vi "Initialize Pressure Transducers.vi"(4 "manifold b":dbl=-51999.8452035158 format="%#_13g", 5 "tube b":dbl=-5165625.86475965 format="%#_13g", 6 "manifold m":dbl=13009471.549307 format="%#_13g", 7 "tube m":dbl=1292765951.79248 format="%#_13g", 8 "error in":errorcluster, 9 "Sensor sample period (ms)":i32=100, 11 "file path":path) -> (0 "Error Out":errorcluster, 3 "task out":refnum<k21>)   [LabVIEW 2018]
uses:
  <vilib>/DAQmx/create/scale.llb/DAQmx Create Scale (Linear).vi
  <vilib>/DAQmx/create/channels.llb/DAQmx Create Channel (AI-Current-Basic).vi
  <vilib>/DAQmx/configure/timing.llb/DAQmx Timing (Sample Clock).vi
  <vilib>/DAQmx/configure/task.llb/DAQmx Configure Logging (TDMS).vi
  <resource>/objmgr/daqmx.rc
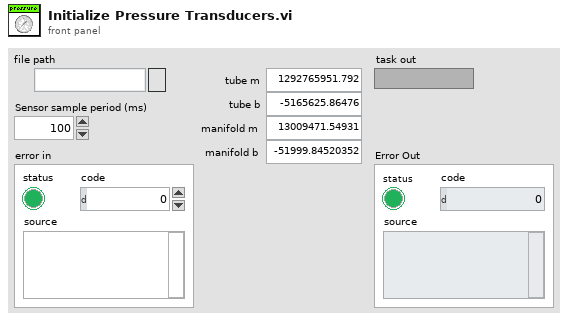
[diagram p1: front panel]
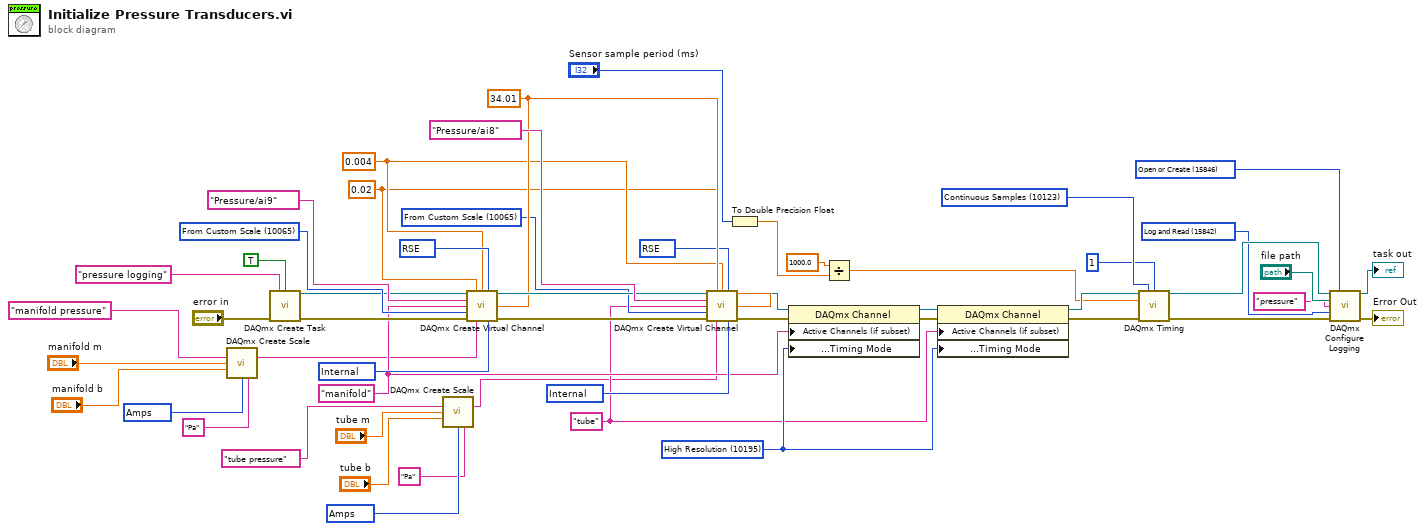
[diagram p0: block diagram]
diagram:
  w10 = 10342 items=["Volts"=10348, "Amps"=10342, "Deg F"=10144, "Deg C"=10143, "Deg R"=10145, "Kelvins"=10325, "Strain"=10299, "Ohms"=10384, "Hz"=10373, "Seconds"=10364, "Meters"=10219, "Inches"=10379, "Degrees"=10146, "Radians"=10273, "Ticks"=10304, "g"=10186, "m/s^2"=12470, "m/s"=15959, "in/s"=15960, "Pascals"=10081, "Newtons"=15875, "Pounds"=15876, "kgf"=15877, "psi"=15879, "bar"=15880, "Nm"=15881, "oz-in"=15882, "lb-in"=15883, "lb-ft"=15884, "Volts/Volt"=15896, "mVolts/Volt"=15897, "pCoulombs"=16103, "Coulombs"=16102, "From TEDS"=12516] ("pre-scaled units")
  w13 = 10342 items=["Volts"=10348, "Amps"=10342, "Deg F"=10144, "Deg C"=10143, "Deg R"=10145, "Kelvins"=10325, "Strain"=10299, "Ohms"=10384, "Hz"=10373, "Seconds"=10364, "Meters"=10219, "Inches"=10379, "Degrees"=10146, "Radians"=10273, "Ticks"=10304, "g"=10186, "m/s^2"=12470, "m/s"=15959, "in/s"=15960, "Pascals"=10081, "Newtons"=15875, "Pounds"=15876, "kgf"=15877, "psi"=15879, "bar"=15880, "Nm"=15881, "oz-in"=15882, "lb-in"=15883, "lb-ft"=15884, "Volts/Volt"=15896, "mVolts/Volt"=15897, "pCoulombs"=16103, "Coulombs"=16102, "From TEDS"=12516] ("pre-scaled units")
  w23 = 15842 items=["Off"=10231, "Log"=15844, "Log and Read"=15842] ("logging mode")
  w24 = 15846 items=["Open"=10437, "Open or Create"=15846, "Create or Replace"=15847, "Create"=15848] ("operation")
  w35 = 10123 items=["Finite Samples"=10178, "Continuous Samples"=10123, "Hardware Timed Single Point"=12522] ("sample mode")
  w38 = 10200 items=["default"=-1, "Internal"=10200, "External"=10167] ("shunt resistor location")
  w39 = 10065 items=["Amps"=10342, "From Custom Scale"=10065] ("units")
  w40 = 10083 items=["default"=-1, "RSE"=10083, "NRSE"=10078, "Differential"=10106, "Pseudodifferential"=12529] ("input terminal configuration")
  w43 = 10195 items=["High Resolution"=10195, "High Speed"=14712, "Best 50 Hz Rejection"=14713, "Best 60 Hz Rejection"=14714] ("ADCTimingMode")
  w18 = "tube" ("name to assign")
  w19 = "manifold" ("name to assign")
  w47 = 34.01 ("external shunt resistor value")
  w46 = 10200 items=["default"=-1, "Internal"=10200, "External"=10167] ("shunt resistor location")
  w52 = 10083 items=["default"=-1, "RSE"=10083, "NRSE"=10078, "Differential"=10106, "Pseudodifferential"=12529] ("input terminal configuration")
  w37 = 0.004 ("minimum value")
  w36 = 0.02 ("maximum value")
  w50 = 10065 items=["Amps"=10342, "From Custom Scale"=10065] ("units")
  n1 = call-poly <vilib>:"DAQmx Create Scale.vi"("name"="manifold pressure", "slope"="manifold m", "y-intercept"="manifold b", "pre-scaled units"=w10, "scaled units"="Pa") -> ("scale out"=w6:tag)  [unwired: 9 in, 1 out]
  n2 = call <vilib>:"DAQmx Create Task.vi"("new task name"="pressure logging", "auto cleanup"=TRUE, "error in"="error in") -> ("task out"=w28:refnum<k21>, "error out"=w29:errorcluster)  [unwired: 11 in]
  n3 = call-poly <vilib>:"DAQmx Create Scale.vi"("name"="tube pressure", "slope"="tube m", "y-intercept"="tube b", "pre-scaled units"=w13, "scaled units"="Pa") -> ("scale out"=w17:tag)  [unwired: 9 in, 1 out]
  n4 = call-poly <vilib>:"DAQmx Create Virtual Channel.vi"("task in"=w28, "maximum value"=w36, "minimum value"=w37, "input terminal configuration"=w52, "physical channels"=tag "Pressure/ai9", "name to assign"=w19, "external shunt resistor value"=w47, "units"=w50, "error in"=w29, "custom scale name"=w6, "shunt resistor location"=w46) -> ("task out"=w48:refnum<k21>, "error out"=w49:errorcluster)  [unwired: 3 in]
  n5 = call-poly <vilib>:"DAQmx Create Virtual Channel.vi"("task in"=w48, "maximum value"=w36, "minimum value"=w37, "input terminal configuration"=w40, "physical channels"=tag "Pressure/ai8", "name to assign"=w18, "external shunt resistor value"=w47, "units"=w39, "error in"=w49, "custom scale name"=w17, "shunt resistor location"=w38) -> ("task out"=w42:refnum<k21>, "error out"=w41:errorcluster)  [unwired: 3 in]
  n6 = To Double Precision Float(number="Sensor sample period (ms)") -> (double precision float=w5:dbl)
  n7 = property on="Property Node" class="DAQmx Channel"(reference=w42, error in=w41, "Active Channels (if subset)"=w19, "Analog Input:General Properties:Digitizer/ADC:Timing Mode"=w43) -> (reference out=w44:refnum<k21>, error out=w45:errorcluster)
  n8 = Divide(x=1000.0, y=w5) -> (x/y=w3:dbl)
  n9 = property on="Property Node" class="DAQmx Channel"(reference=w44, error in=w45, "Active Channels (if subset)"=w18, "Analog Input:General Properties:Digitizer/ADC:Timing Mode"=w43) -> (reference out=w32:refnum<k21>, error out=w33:errorcluster)
  n10 = call-poly <vilib>:"DAQmx Timing.vi"("task/channels in"=w32, "sample mode"=w35, "samples per channel"=1 ("number of samples"), "rate"=w3, "error in"=w33) -> ("task out"=w26:refnum<k21>, "error out"=w27:errorcluster)  [unwired: 9 in]
  n11 = call-poly <vilib>:"DAQmx Configure Logging.vi"("task/channels in"=w26, "operation"=w24, "file path"="file path", "group name"="pressure", "logging mode"=w23, "error in"=w27) -> ("task out"=→"task out":refnum<k21>, "error out"=→"Error Out":errorcluster)  [unwired: 8 in]
